vi "SVX9000App.vi"() -> ()   [LabVIEW 2011]
panel:
  in  "Execute Profile":bool
  in  "Change Profile":u8(ring) items=["Select a Profile", "Closing Profile", "Opening Profile"]
  out "SVX Freq":dbl(graph)
  in  "Ramp":sgl=10.0 min=0 max=10 step=0.1 format="%.1f"
  in  "Ramp Shape":bool
  in  "Dec Time":sgl=30.0 min=0 max=6553.5 step=0.1 format="%.1f"
  in  "Decceleration Time":bool
  in  "Acc Time":sgl=30.0 min=0 max=6553.5 step=0.1 format="%.1f"
  in  "Acceleration Time":bool
  in  "left":bool
  in  "right":bool
  in  "Vel %":u8=100 max=100 step=1
  in  "Velocity":bool
  in  "Device ID":u8=255 min=1 step=1
  in  "stop":bool
  in  "start":bool
  in  "Remote port":u16=502
  in  "Server address":string="192.168.1.3"
  in  "stop_app":bool
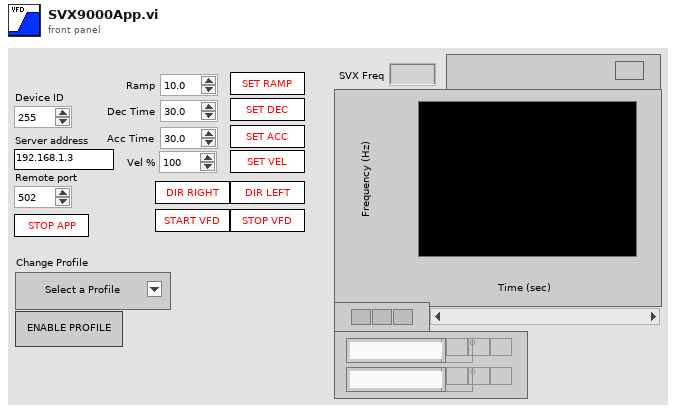
[diagram p1: front panel]
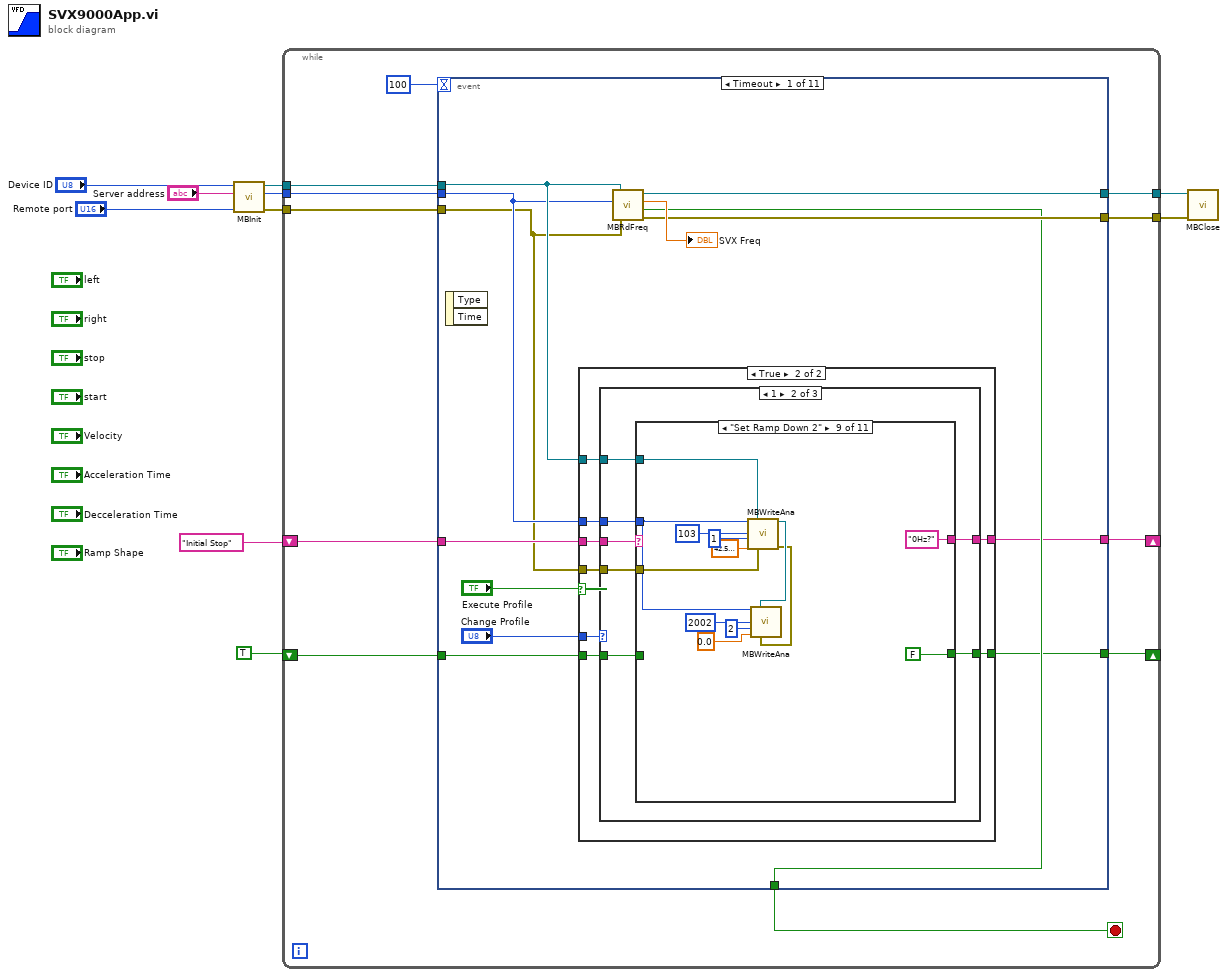
[diagram p0: block diagram]
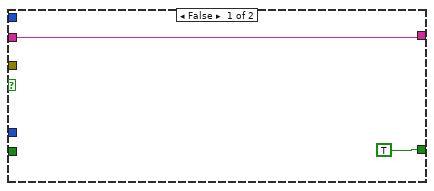
[diagram p2: hidden frame]
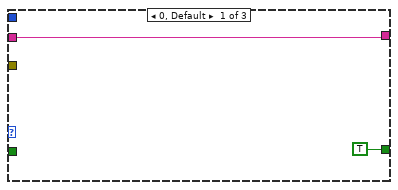
[diagram p3: hidden frame]
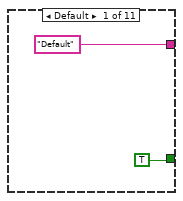
[diagram p4: hidden frame]
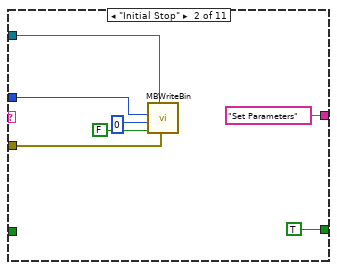
[diagram p5: hidden frame]
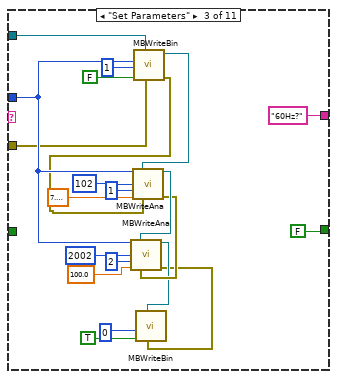
[diagram p6: hidden frame]
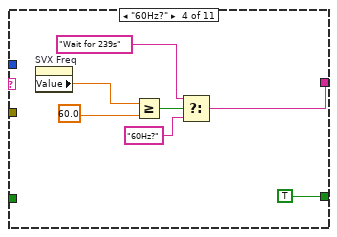
[diagram p7: hidden frame]
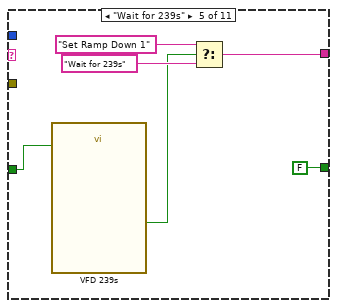
[diagram p8: hidden frame]
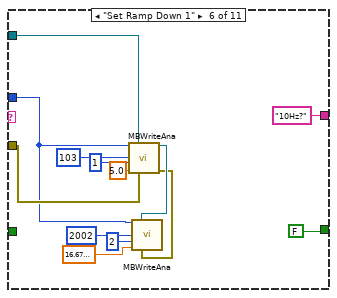
[diagram p9: hidden frame]
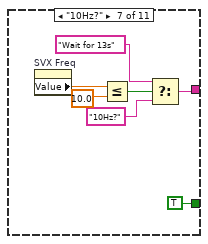
[diagram p10: hidden frame]
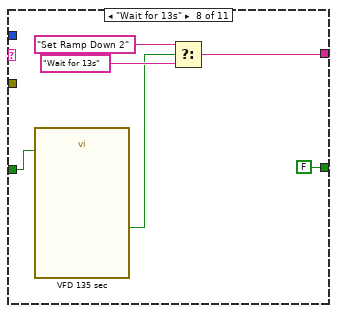
[diagram p11: hidden frame]
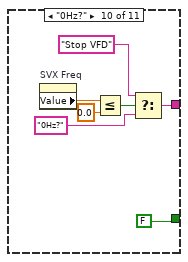
[diagram p12: hidden frame]
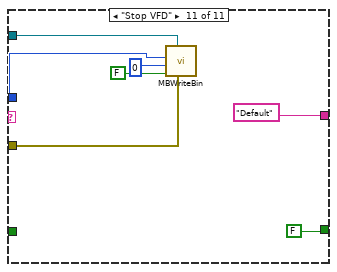
[diagram p13: hidden frame]
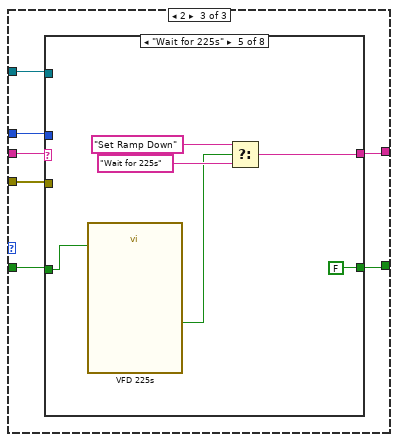
[diagram p14: hidden frame]
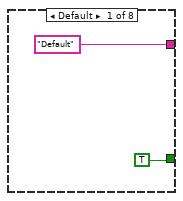
[diagram p15: hidden frame]
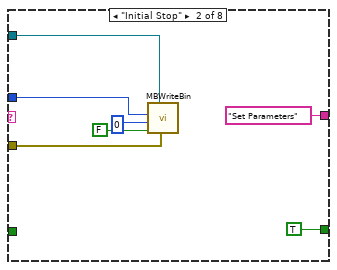
[diagram p16: hidden frame]
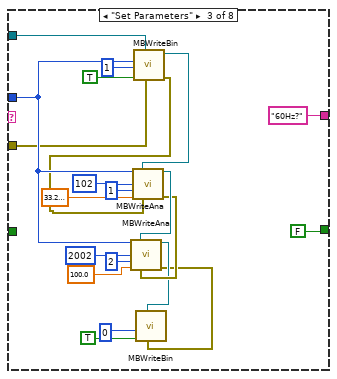
[diagram p17: hidden frame]
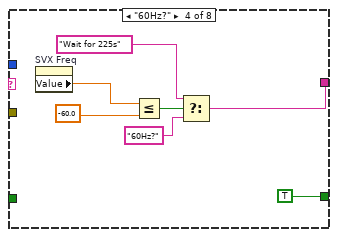
[diagram p18: hidden frame]
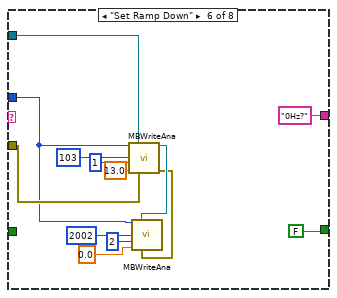
[diagram p19: hidden frame]
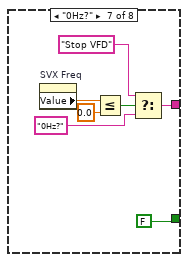
[diagram p20: hidden frame]
diagram:
  n1 = call "MBInit.vi"("Remote port"="Remote port", "Server address"="Server address", "Device ID"="Device ID") -> ("error out"=w9:errorcluster, "Device ID"=w6:u8, "TCP Network Connection out"=w10:refnum<k5>)  [unwired: 6 in]
  n2 = while {
    tunnel: w9 -> [w17]
    tunnel: w10 -> [w19]
    tunnel: w6 -> [w18]
    tunnel: [w21] -> w4
    tunnel: [w20] -> w3
    shift-right: [w13] -> _
    shift-left: "Initial Stop" -> [w14]
    shift-right: [w12] -> _
    shift-left: TRUE -> [w11]
    stop <- w16 stop-if-true
    n3 = event shown="[0] Timeout" {
      selector: _ -> [_ _ _ _ _ _ _ _ _ _ _]
      dyn-events: _ -> [_ _ _ _ _ _ _ _ _ _ _]
      timeout: 100 -> [_ _ _ _ _ _ _ _ _ _ _]
      tunnel: w19 -> [w26 w230 w236 w241 w251 w261 w270 w276 w284 w294 w306]
      tunnel: w18 -> [w25 _ w235 w242 w252 w260 w269 w277 w285 w293 w305]
      tunnel: w17 -> [w24 w229 w234 w245 w250 w259 w268 w278 w286 w292 w304]
      tunnel: [w33 w229 w233 w244 w254 w263 w271 w279 w287 w296 w303] -> w21
      tunnel: [w32 w230 w232 w243 w253 w262 w272 w280 w288 w295 w302] -> w20
      tunnel: [w31 FALSE ("Error Flag") w231 w240 w249 w258 w267 w275 w283 w291 w299] -> w16
      tunnel: w14 -> [w30 _ _ _ _ _ _ _ _ _ _]
      tunnel: [w29 "Initial Stop" _ _ _ _ _ _ _ _ _] -> w13
      tunnel: [w23 _ _ _ _ _ _ _ _ _ _] -> w12
      tunnel: w11 -> [w22 _ _ _ _ _ _ _ _ _ _]
      event Timeout {
        n4 = event-data() -> ()  [unwired: 1 in, 2 out]
        n5 = case shown="True" "Execute Profile" {
          tunnel: w30 -> [w36 w44]
          tunnel: [w36 w43] -> w29
          tunnel: "Change Profile" -> [_ w42]
          tunnel: w26 -> [_ w41]
          tunnel: w25 -> [_ w40]
          tunnel: w24 -> [_ w39]
          tunnel: [TRUE w38] -> w23
          tunnel: w22 -> [_ w37]
          frame False {
          }
          frame True {
            n6 = case shown="1" w42 {
              tunnel: w44 -> [w46 w53 w154]
              tunnel: [w46 w52 w151] -> w43
              tunnel: w41 -> [_ w51 w156]
              tunnel: w40 -> [_ w50 w155]
              tunnel: w39 -> [_ w49 w153]
              tunnel: [TRUE w48 w150] -> w38
              tunnel: w37 -> [_ w47 w152]
              frame 0, Default {
              }
              frame 1 {
                n7 = case shown="\"Set Ramp Down 2\"" w53 {
                  tunnel: ["Default" "Set Parameters" "60Hz?" w86 w93 "10Hz?" w113 w119 "0Hz?" w138 "Default"] -> w52
                  tunnel: w51 -> [_ w59 w71 _ _ w103 _ _ w129 _ w146]
                  tunnel: w50 -> [_ w58 w74 _ _ w101 _ _ w127 _ w145]
                  tunnel: w49 -> [_ w57 w70 _ _ w102 _ _ w128 _ w144]
                  tunnel: [TRUE TRUE FALSE TRUE FALSE FALSE TRUE FALSE FALSE FALSE FALSE] -> w48
                  tunnel: w47 -> [_ _ _ _ w92 _ _ w117 _ _ _]
                  frame Default {
                  }
                  frame "Initial Stop" {
                    n8 = call "MBWriteBin.vi"("error in"=w57, "NetRefTCP in"=w59, "Bit"=FALSE, "MB Reg No"=u8 0, "Device ID"=w58) -> ()  [unwired: 3 in, 3 out]
                  }
                  frame "Set Parameters" {
                    n9 = call "MBWriteBin.vi"("error in"=w70, "NetRefTCP in"=w71, "Bit"=FALSE, "MB Reg No"=u8 1, "Device ID"=w74) -> ("error out"=w69:errorcluster, "NetRefTCP out"=w68:refnum<k5>)  [unwired: 3 in, 1 out]
                    n10 = call "MBWriteAna.vi"("Device ID"=w74, "NetRefTCP in"=w68, "MB Reg No"=u16 102 ("Word address"), "Scale"=u8 1, "Value"=sgl 7.1, "error in"=w69) -> ("NetRefTCP out"=w67:refnum<k5>, "error out"=w66:errorcluster)  [unwired: 7 in, 1 out]
                    n11 = call "MBWriteAna.vi"("Device ID"=w74, "NetRefTCP in"=w67, "MB Reg No"=u16 2002, "Scale"=u8 2, "Value"=sgl 100.0, "error in"=w66) -> ("NetRefTCP out"=w65:refnum<k5>, "error out"=w64:errorcluster)  [unwired: 7 in, 1 out]
                    n12 = call "MBWriteBin.vi"("error in"=w64, "NetRefTCP in"=w65, "Bit"=TRUE, "MB Reg No"=u8 0) -> ()  [unwired: 4 in, 3 out]
                  }
                  frame "60Hz?" {
                    n13 = property on="SVX Freq" class="WFChart (strict)"() -> ("Value"=w85:dbl)  [unwired: 2 in, 2 out]
                    n14 = Greater Or Equal?(x=w85, y=60.0 ("f")) -> (x >= y?=w89:bool)
                    n15 = Select(t="Wait for 239s", s=w89, f="60Hz?") -> (s? t:f=w86:string)
                  }
                  frame "Wait for 239s" {
                    n16 = call "VFD 239s"("Reset"=w92) -> ("Time has Elapsed"=w94:bool)  [unwired: 11 in, 7 out]
                    n17 = Select(t="Set Ramp Down 1", s=w94, f="Wait for 239s") -> (s? t:f=w93:string)
                  }
                  frame "Set Ramp Down 1" {
                    n18 = call "MBWriteAna.vi"("Device ID"=w101, "NetRefTCP in"=w103, "MB Reg No"=u16 103 ("Word address"), "Scale"=u8 1, "Value"=sgl 5.0, "error in"=w102) -> ("NetRefTCP out"=w99:refnum<k5>, "error out"=w98:errorcluster)  [unwired: 7 in, 1 out]
                    n19 = call "MBWriteAna.vi"("Device ID"=w101, "NetRefTCP in"=w99, "MB Reg No"=u16 2002, "Scale"=u8 2, "Value"=sgl 16.67, "error in"=w98) -> ()  [unwired: 7 in, 3 out]
                  }
                  frame "10Hz?" {
                    n20 = property on="SVX Freq" class="WFChart (strict)"() -> ("Value"=w112:dbl)  [unwired: 2 in, 2 out]
                    n21 = Less Or Equal?(x=w112, y=10.0 ("f")) -> (x <= y?=w116:bool)
                    n22 = Select(t="Wait for 13s", s=w116, f="10Hz?") -> (s? t:f=w113:string)
                  }
                  frame "Wait for 13s" {
                    n23 = call "VFD 135 sec"("Reset"=w117) -> ("Time has Elapsed"=w120:bool)  [unwired: 11 in, 7 out]
                    n24 = Select(t="Set Ramp Down 2", s=w120, f="Wait for 13s") -> (s? t:f=w119:string)
                  }
                  frame "Set Ramp Down 2" {
                    n25 = call "MBWriteAna.vi"("Device ID"=w127, "NetRefTCP in"=w129, "MB Reg No"=u16 103 ("Word address"), "Scale"=u8 1, "Value"=sgl 42.6, "error in"=w128) -> ("NetRefTCP out"=w126:refnum<k5>, "error out"=w125:errorcluster)  [unwired: 7 in, 1 out]
                    n26 = call "MBWriteAna.vi"("Device ID"=w127, "NetRefTCP in"=w126, "MB Reg No"=u16 2002, "Scale"=u8 2, "Value"=sgl 0.0, "error in"=w125) -> ()  [unwired: 7 in, 3 out]
                  }
                  frame "0Hz?" {
                    n27 = property on="SVX Freq" class="WFChart (strict)"() -> ("Value"=w137:dbl)  [unwired: 2 in, 2 out]
                    n28 = Less Or Equal?(x=w137, y=0.0 ("f")) -> (x <= y?=w141:bool)
                    n29 = Select(t="Stop VFD", s=w141, f="0Hz?") -> (s? t:f=w138:string)
                  }
                  frame "Stop VFD" {
                    n30 = call "MBWriteBin.vi"("error in"=w144, "NetRefTCP in"=w146, "Bit"=FALSE, "MB Reg No"=u8 0, "Device ID"=w145) -> ()  [unwired: 3 in, 3 out]
                  }
                }
              }
              frame 2 {
                n31 = case shown="\"Wait for 225s\"" w154 {
                  tunnel: ["Default" "Set Parameters" "60Hz?" w189 w196 "0Hz?" w215 "Default"] -> w151
                  tunnel: w156 -> [_ w162 w174 _ _ w206 _ w223]
                  tunnel: w155 -> [_ w161 w177 _ _ w204 _ w222]
                  tunnel: w153 -> [_ w160 w173 _ _ w205 _ w221]
                  tunnel: [TRUE TRUE FALSE TRUE FALSE FALSE FALSE FALSE] -> w150
                  tunnel: w152 -> [_ _ _ _ w195 _ _ _]
                  frame Default {
                  }
                  frame "Initial Stop" {
                    n32 = call "MBWriteBin.vi"("error in"=w160, "NetRefTCP in"=w162, "Bit"=FALSE, "MB Reg No"=u8 0, "Device ID"=w161) -> ()  [unwired: 3 in, 3 out]
                  }
                  frame "Set Parameters" {
                    n33 = call "MBWriteBin.vi"("error in"=w173, "NetRefTCP in"=w174, "Bit"=TRUE, "MB Reg No"=u8 1, "Device ID"=w177) -> ("error out"=w172:errorcluster, "NetRefTCP out"=w171:refnum<k5>)  [unwired: 3 in, 1 out]
                    n34 = call "MBWriteAna.vi"("Device ID"=w177, "NetRefTCP in"=w171, "MB Reg No"=u16 102 ("Word address"), "Scale"=u8 1, "Value"=sgl 33.3, "error in"=w172) -> ("NetRefTCP out"=w170:refnum<k5>, "error out"=w169:errorcluster)  [unwired: 7 in, 1 out]
                    n35 = call "MBWriteAna.vi"("Device ID"=w177, "NetRefTCP in"=w170, "MB Reg No"=u16 2002, "Scale"=u8 2, "Value"=sgl 100.0, "error in"=w169) -> ("NetRefTCP out"=w168:refnum<k5>, "error out"=w167:errorcluster)  [unwired: 7 in, 1 out]
                    n36 = call "MBWriteBin.vi"("error in"=w167, "NetRefTCP in"=w168, "Bit"=TRUE, "MB Reg No"=u8 0) -> ()  [unwired: 4 in, 3 out]
                  }
                  frame "60Hz?" {
                    n37 = property on="SVX Freq" class="WFChart (strict)"() -> ("Value"=w188:dbl)  [unwired: 2 in, 2 out]
                    n38 = Less Or Equal?(x=w188, y=-60.0 ("f")) -> (x <= y?=w192:bool)
                    n39 = Select(t="Wait for 225s", s=w192, f="60Hz?") -> (s? t:f=w189:string)
                  }
                  frame "Wait for 225s" {
                    n40 = call "VFD 225s"("Reset"=w195) -> ("Time has Elapsed"=w197:bool)  [unwired: 11 in, 7 out]
                    n41 = Select(t="Set Ramp Down", s=w197, f="Wait for 225s") -> (s? t:f=w196:string)
                  }
                  frame "Set Ramp Down" {
                    n42 = call "MBWriteAna.vi"("Device ID"=w204, "NetRefTCP in"=w206, "MB Reg No"=u16 103 ("Word address"), "Scale"=u8 1, "Value"=sgl 13.0, "error in"=w205) -> ("NetRefTCP out"=w202:refnum<k5>, "error out"=w201:errorcluster)  [unwired: 7 in, 1 out]
                    n43 = call "MBWriteAna.vi"("Device ID"=w204, "NetRefTCP in"=w202, "MB Reg No"=u16 2002, "Scale"=u8 2, "Value"=sgl 0.0, "error in"=w201) -> ()  [unwired: 7 in, 3 out]
                  }
                  frame "0Hz?" {
                    n44 = property on="SVX Freq" class="WFChart (strict)"() -> ("Value"=w214:dbl)  [unwired: 2 in, 2 out]
                    n45 = Less Or Equal?(x=w214, y=0.0 ("f")) -> (x <= y?=w218:bool)
                    n46 = Select(t="Stop VFD", s=w218, f="0Hz?") -> (s? t:f=w215:string)
                  }
                  frame "Stop VFD" {
                    n47 = call "MBWriteBin.vi"("error in"=w221, "NetRefTCP in"=w223, "Bit"=FALSE, "MB Reg No"=u8 0, "Device ID"=w222) -> ()  [unwired: 3 in, 3 out]
                  }
                }
              }
            }
          }
        }
        n48 = call "MBRdFreq.vi"("error in"=w24, "Device ID"=w25, "NetRefTCP in"=w26) -> ("error out"=w33:errorcluster, "Error Flag"=w31:bool, "Frequency"=→"SVX Freq":dbl, "NetRefTCP out"=w32:refnum<k5>)  [unwired: 1 in]
      }
      event "Change Profile": Value Change {
        n49 = event-data() -> ()  [unwired: 1 in, 5 out]
      }
      event "Velocity": Value Change {
        n50 = event-data() -> ()  [unwired: 1 in, 5 out]
        n51 = call "MBWriteAna.vi"("Device ID"=w235, "NetRefTCP in"=w236, "MB Reg No"=u16 2002, "Scale"=u8 2, "Value"="Vel %", "error in"=w234) -> ("NetRefTCP out"=w232:refnum<k5>, "Error Flag"=w231:bool, "error out"=w233:errorcluster)  [unwired: 7 in]
      }
      event "Acceleration Time": Value Change {
        n52 = event-data() -> ()  [unwired: 1 in, 5 out]
        n53 = call "MBWriteAna.vi"("Device ID"=w242, "NetRefTCP in"=w241, "MB Reg No"=u16 102 ("Word address"), "Scale"=u8 1, "Value"="Acc Time", "error in"=w245) -> ("NetRefTCP out"=w243:refnum<k5>, "Error Flag"=w240:bool, "error out"=w244:errorcluster)  [unwired: 7 in]
      }
      event "Decceleration Time": Value Change {
        n54 = event-data() -> ()  [unwired: 1 in, 5 out]
        n55 = call "MBWriteAna.vi"("Device ID"=w252, "NetRefTCP in"=w251, "MB Reg No"=u16 103 ("Word address"), "Scale"=u8 1, "Value"="Dec Time", "error in"=w250) -> ("NetRefTCP out"=w253:refnum<k5>, "Error Flag"=w249:bool, "error out"=w254:errorcluster)  [unwired: 7 in]
      }
      event "Ramp Shape": Value Change {
        n56 = event-data() -> ()  [unwired: 1 in, 5 out]
        n57 = call "MBWriteAna.vi"("Device ID"=w260, "NetRefTCP in"=w261, "MB Reg No"=u16 499 ("Word address"), "Scale"=u8 1, "Value"="Ramp", "error in"=w259) -> ("NetRefTCP out"=w262:refnum<k5>, "Error Flag"=w258:bool, "error out"=w263:errorcluster)  [unwired: 7 in]
      }
      event "left": Value Change {
        n58 = event-data() -> ()  [unwired: 1 in, 5 out]
        n59 = call "MBWriteBin.vi"("error in"=w268, "NetRefTCP in"=w270, "Bit"=TRUE, "MB Reg No"=u8 1, "Device ID"=w269) -> ("error out"=w271:errorcluster, "Error Flag"=w267:bool, "NetRefTCP out"=w272:refnum<k5>)  [unwired: 3 in]
      }
      event "right": Value Change {
        n60 = event-data() -> ()  [unwired: 1 in, 5 out]
        n61 = call "MBWriteBin.vi"("error in"=w278, "NetRefTCP in"=w276, "Bit"=FALSE, "MB Reg No"=u8 1, "Device ID"=w277) -> ("error out"=w279:errorcluster, "Error Flag"=w275:bool, "NetRefTCP out"=w280:refnum<k5>)  [unwired: 3 in]
      }
      event "stop": Value Change {
        n62 = event-data() -> ()  [unwired: 1 in, 5 out]
        n63 = call "MBWriteBin.vi"("error in"=w286, "NetRefTCP in"=w284, "Bit"=FALSE, "MB Reg No"=u8 0, "Device ID"=w285) -> ("error out"=w287:errorcluster, "Error Flag"=w283:bool, "NetRefTCP out"=w288:refnum<k5>)  [unwired: 3 in]
      }
      event "start": Value Change {
        n64 = event-data() -> ()  [unwired: 1 in, 5 out]
        n65 = call "MBWriteBin.vi"("error in"=w292, "NetRefTCP in"=w294, "Bit"=TRUE, "MB Reg No"=u8 0, "Device ID"=w293) -> ("error out"=w296:errorcluster, "Error Flag"=w291:bool, "NetRefTCP out"=w295:refnum<k5>)  [unwired: 3 in]
      }
      event "stop_app": Value Change {
        n66 = event-data() -> ()  [unwired: 1 in, 5 out]
        n67 = call "MBWriteBin.vi"("error in"=w304, "NetRefTCP in"=w306, "Bit"=FALSE, "MB Reg No"=u8 0, "Device ID"=w305) -> ("error out"=w303:errorcluster, "Error Flag"=w301:bool, "NetRefTCP out"=w302:refnum<k5>)  [unwired: 3 in]
        n68 = Or(x=w301, y="stop_app") -> (x .or. y?=w299:bool)
      }
    }
  }
  n69 = call "MBClose.vi"("error in (no error)"=w4, "TCP Network Connection in"=w3) -> ()  [unwired: 10 in]
